vi "Byte Buffer.Mapping.Read.vi"(8 "error in (no error)":errorcluster, 9 "initial buffer count (100)":i32=100, 10 "mappings":T1[](array[typedef]), 11 "Byte Buffer in":refnum<class "Byte Buffer.lvclass">) -> (0 "error out":errorcluster, 2 "mappings dup":T1[](array[typedef]), 3 "Byte Buffer out":refnum<class "Byte Buffer.lvclass">)   [LabVIEW 2016, in "VeriStand Data.lvlib" / "Byte Buffer.lvclass"]
uses:
  Byte Buffer.lvclass
  Byte Buffer.Mapping.ctl
  Typedefs/Typedefs.Data Types.ctl
  Byte Buffer.lvclass/Byte Buffer.ctl
  SubVIs/Sizeof.Array.vi
  Byte Buffer.Read.vi
  Byte Buffer.Read (1D Boolean).vi
  Type Conversion/Type Conversion.To Double.Subset.vi
  Type Conversion/Type Conversion.To Double.Subset (1D Boolean).vi
  Byte Buffer.Read (1D SGL).vi
  Type Conversion/Type Conversion.To Double.Subset (1D SGL).vi
  Byte Buffer.Read (1D DBL).vi
  Byte Buffer.Read (1D I8).vi
  Type Conversion/Type Conversion.To Double.Subset (1D I8).vi
  Byte Buffer.Read (1D I16).vi
  Type Conversion/Type Conversion.To Double.Subset (1D I16).vi
  Byte Buffer.Read (1D I32).vi
  Type Conversion/Type Conversion.To Double.Subset (1D I32).vi
  Byte Buffer.Read (1D I64).vi
  Type Conversion/Type Conversion.To Double.Subset (1D I64).vi
  Byte Buffer.Read (1D U8).vi
  Type Conversion/Type Conversion.To Double.Subset (1D U8).vi
  Byte Buffer.Read (1D U16).vi
  Type Conversion/Type Conversion.To Double.Subset (1D U16).vi
  Byte Buffer.Read (1D U32).vi
  Type Conversion/Type Conversion.To Double.Subset (1D U32).vi
  Byte Buffer.Read (1D U64).vi
  Type Conversion/Type Conversion.To Double.Subset (1D U64).vi
  SubVIs/Sizeof.Scalar.vi
  Type Conversion/Type Conversion.To Double.vi
  Type Conversion/Type Conversion.To Double (1D Boolean).vi
  Type Conversion/Type Conversion.To Double (1D SGL).vi
  Type Conversion/Type Conversion.To Double (1D I8).vi
  Type Conversion/Type Conversion.To Double (1D I16).vi
  Type Conversion/Type Conversion.To Double (1D I32).vi
  Type Conversion/Type Conversion.To Double (1D I64).vi
  Type Conversion/Type Conversion.To Double (1D U8).vi
  Type Conversion/Type Conversion.To Double (1D U16).vi
  Type Conversion/Type Conversion.To Double (1D U32).vi
  Type Conversion/Type Conversion.To Double (1D U64).vi
  Memory Management/Memory Management.Handle Return.vi
  VeriStand Data.lvlib
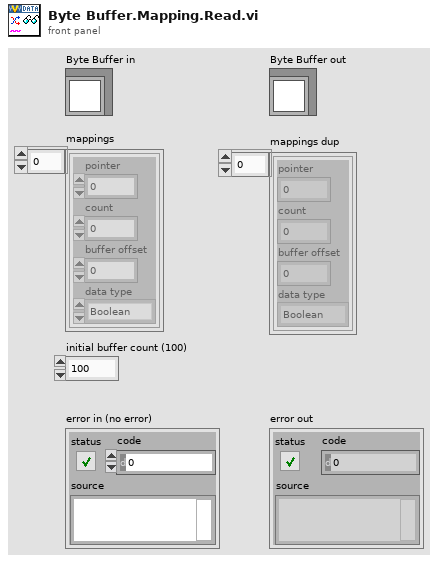
[diagram p1: front panel]
types:
  T1 = typedef "VeriStand Data.lvlib/Byte Buffer.lvclass/Byte Buffer.Mapping.ctl" = cluster{"pointer":u64, "count":i32, "buffer offset":i32, "data type":T2}
  T2 = typedef "VeriStand Data.lvlib/Typedefs.Data Types.ctl" = enum16{"Boolean", "Single", "Double", "I8", "I16", "I32", "I64", "U8", "U16", "U32", "U64"}
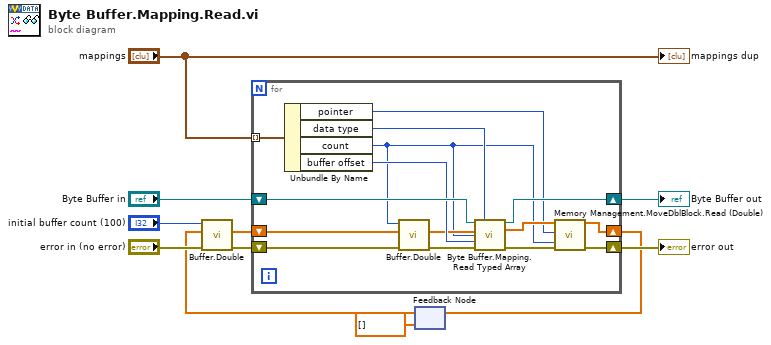
[diagram p0: block diagram]
diagram:
  n1 = feedback #1(dbl[] [] ("src out")) -> (w2:dbl[])
  n2 = call "Buffer.Double.vi"("error in (no error)"="error in (no error)", "buffer in"=w2, "minimum size"="initial buffer count (100)") -> ("error out"=w4:errorcluster, "buffer out"=w3:dbl[])  [unwired: 7 in]
  n3 = for {
    tunnel: "mappings" -> [w25] mode=indexing
    shift-right: [w20] -> w11
    shift-left: w4 -> [w16]
    shift-right: [w23] -> w9
    shift-left: "Byte Buffer in" -> [w26]
    shift-right: [w18] -> w8
    shift-left: w3 -> [w15]
    n4 = Unbundle By Name(w25) -> ("pointer"=w17:u64, "data type"=w22:T2, "count"=w12:i32, "buffer offset"=w24:i32)
    n5 = call "Buffer.Double.vi"("error in (no error)"=w16, "buffer in"=w15, "minimum size"=w12) -> ("error out"=w14:errorcluster, "buffer out"=w13:dbl[])  [unwired: 7 in]
    n6 = call "Byte Buffer.Mapping.Read Typed Array.vi"("Byte Buffer in"=w26, "data type"=w22, "buffer in"=w13, "count"=w12, "buffer offset"=w24, "error in (no error)"=w14) -> ("Byte Buffer out"=w23:refnum<class "Byte Buffer.lvclass">, "buffer out"=w19:dbl[], "error out"=w21:errorcluster)  [unwired: 6 in, 1 out]
    n7 = call "Memory Management.MoveDblBlock.Read (Double).vi"("src in"=w19, "dst ptr in"=w17, "count"=w12, "error in (no error)"=w21) -> ("src out"=w18:dbl[], "error out"=w20:errorcluster)  [unwired: 10 in, 4 out]
  }
  "error out" <- w11
  "Byte Buffer out" <- w9
  n8 = feedback-in #1(w8) -> ()
  "mappings dup" <- "mappings"
